vi "Get HUE.vi"(8 "error in (no error)":errorcluster caption="entrée d'erreur (pas d'erreur)", 11 "Class Instrument LED_Analyser en entrée":refnum<class "Class Instrument LED_Analyser.lvclass">) -> (0 "error out":errorcluster caption="sortie d'erreur", 2 "HUE":dbl format="%#.6f", 3 "Class Instrument LED_Analyser en sortie":refnum<class "Class Instrument LED_Analyser.lvclass">)   [LabVIEW 2020, in "Library Instrument & Equipement.lvlib" / "Library Instruments.lvlib" / "Class Instrument LED_Analyser.lvclass"]
uses:
  Class Instrument LED_Analyser.lvclass
  Class Instrument LED_Analyser.lvclass/Class Instrument LED_Analyser.ctl
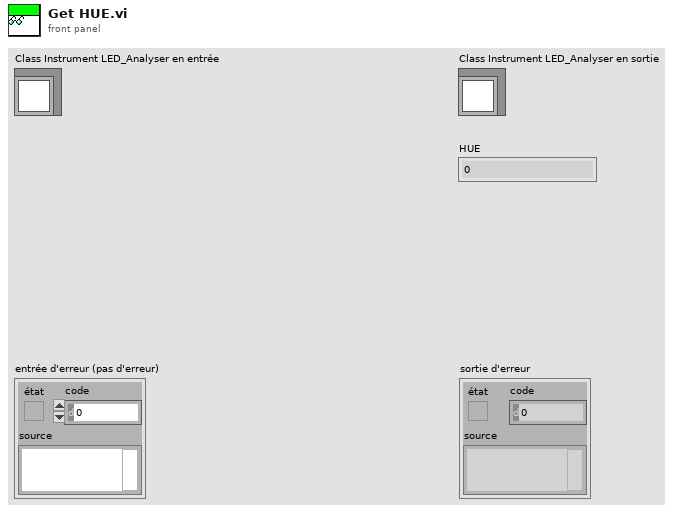
[diagram p1: front panel]
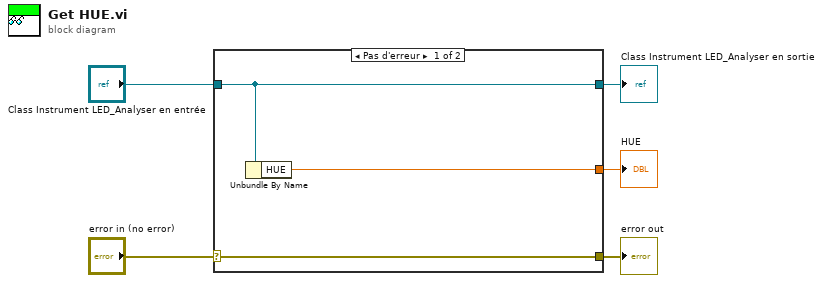
[diagram p0: block diagram]
diagram:
  n1 = case shown="Pas d'erreur" "error in (no error)" {
    selector: "error in (no error)" -> [w8 w9]
    tunnel: [w8 w9] -> w4
    tunnel: [w7 w10] -> w2
    tunnel: "Class Instrument LED_Analyser en entrée" -> [w7 w10]
    tunnel: [w6 _] -> w1
    frame No Error {
      n2 = Unbundle By Name(w7) -> ("HUE"=w6:dbl)
    }
    frame Error {
    }
  }
  "error out" <- w4
  "Class Instrument LED_Analyser en sortie" <- w2
  "HUE" <- w1
